vi "Launch PID Loop.vi"(8 "error in (no error)":errorcluster, 11 "PID Loop in":refnum<class "PID Loop.lvclass">) -> (0 "error out":errorcluster, 2 "Message Queue":refnum<queue>)   [LabVIEW 2024, in "PID Loop.lvlib" / "PID Loop.lvclass"]
uses:
  PID Loop.lvclass
  OOQMH/Message/Message.lvclass
  C:/Users/uspoaotto/OneDrive - Oregon Tool/Desktop/working copies/helperLoop/src/OOQMH/OOQMH/OOQMH.lvclass
  OOQMH/OOQMH/OOQMH.lvclass
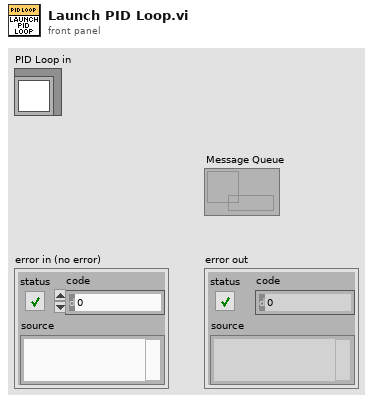
[diagram p1: front panel]
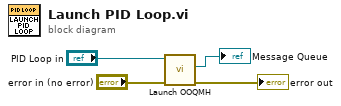
[diagram p0: block diagram]
diagram:
  n1 = call "Launch OOQMH.vi"("error in (no error)"="error in (no error)", "OOQMH in"="PID Loop in") -> ("error out"=→"error out":errorcluster, "Message Queue"=→"Message Queue":refnum<queue>)  [unwired: 8 in]
